vi "PH_gentec_P-Link.ProcPeriodic.vi"(0 "i ref in":refnum<vi>, 3 "ms timeout (100)":i32=100, 5 "error in (no error)":errorcluster) -> (14 "i ref out":refnum<vi>, 17 "timed out":bool, 19 "error out":errorcluster)   [LabVIEW 2014, in "PH_gentec_P-Link.lvlib"]
doc: "This method serves to periodically do things. In this case, it reads the current value from the powermeter. If the Start Stop - value is true, the statistic data is read out as well. Finally, these data is send to own attributes and the GUI elements."
uses:
  PH_gentec_P-Link.lvlib
  PH_Basics/PH_Powermeter_BaseClass/PH_Powermeter_BaseClass.lvlib
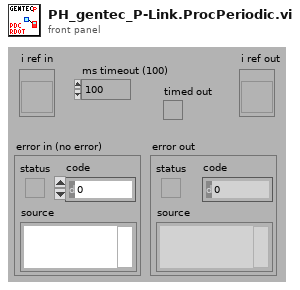
[diagram p1: front panel]
types:
  T1 = typedef "PH_Powermeter_BaseClass.lvlib/PH_Powermeter_BaseClass.State.ctl" = enum32{"off", "operating", "opened", "checked", "connected", "Sets to change", "running"}
  T2 = typedef "PH_gentec_P-Link.lvlib/PH_gentec_P-Link.i attribute.ctl" = cluster{"GUI References":cluster{"Wanted Head Settings":refnum<vi>, "Current Head Settings":refnum<vi>, "Set Auto Range":refnum<vi>, "Trigger Polarity":refnum<vi>, "Trigger Source":refnum<vi>, "Waveform Averages":refnum<vi>, "Continuous":refnum<vi>, "get one Value":refnum<vi>, "Set Zero":refnum<vi>}, "Wanted Head Settings":T3, "Current Head Settings":T3}
  T3 = typedef "PH_gentec_P-Link.lvlib/PH_gentec_P-Link.Head Settings.ctl" = cluster{"Enable Anticipation":bool, "Set Auto Range":bool, "Set Zero":i32, "Current":i32, "Start Data Flow":bool}
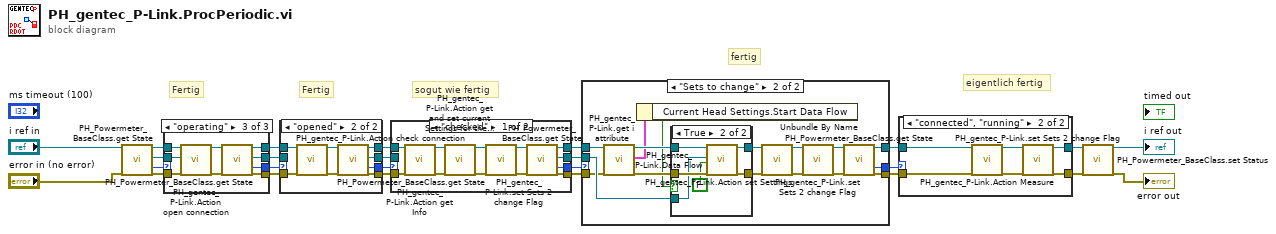
[diagram p0: block diagram]
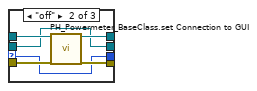
[diagram p8: hidden frame]
diagram:
  # "eigentlich fertig"
  # "fertig"
  # "sogut wie fertig"
  # "Fertig"
  # "Fertig"
  n1 = call "PH_Powermeter_BaseClass.get State.vi"("VI in"="i ref in", "error in (no error)"="error in (no error)") -> ("VI out"=w24:refnum<vi>, "VISA resource"=w23:refnum<visa-resource-name>, "State"=w18:T1, "error out"=w25:errorcluster)  [unwired: 14 in]
  n2 = case shown="\"operating\"" w18 {
    selector: w18 -> [w27 w30 _]
    tunnel: w25 -> [w29 w34 w44]
    tunnel: [w29 w32 w40] -> w16
    tunnel: w23 -> [w28 w31 w43]
    tunnel: [w28 w31 w37] -> w14
    tunnel: [w27 w30 w36] -> w15
    tunnel: w24 -> [w26 w35 w42]
    tunnel: [w26 w33 w38] -> w17
    frame Default {
    }
    frame "off" {
      n3 = call "PH_Powermeter_BaseClass.set Connection to GUI.vi"("i ref in"=w35, "error in"=w34) -> ("i ref out"=w33:refnum<vi>, "error out"=w32:errorcluster)  [unwired: 16 in]
    }
    frame "operating" {
      n4 = call "PH_gentec_P-Link.Action open connection.vi"("i ref in"=w42, "VISA resource in"=w43, "error in"=w44) -> ("i ref out"=w39:refnum<vi>, "error out"=w41:errorcluster)  [unwired: 15 in]
      n5 = call "PH_Powermeter_BaseClass.get State.vi"("VI in"=w39, "error in (no error)"=w41) -> ("VI out"=w38:refnum<vi>, "VISA resource"=w37:refnum<visa-resource-name>, "State"=w36:T1, "error out"=w40:errorcluster)  [unwired: 14 in]
    }
  }
  n6 = case shown="\"opened\"" w15 {
    selector: w15 -> [w46 _]
    tunnel: w16 -> [w48 w49]
    tunnel: [w48 w54] -> w12
    tunnel: w14 -> [w47 _]
    tunnel: [w47 w51] -> w10
    tunnel: [w46 w50] -> w11
    tunnel: w17 -> [w45 w56]
    tunnel: [w45 w52] -> w13
    frame Default {
    }
    frame "opened" {
      n7 = call "PH_gentec_P-Link.Action check connection.vi"("i ref in"=w56, "error in"=w49) -> ("i ref out"=w53:refnum<vi>, "error out"=w55:errorcluster)  [unwired: 16 in]
      n8 = call "PH_Powermeter_BaseClass.get State.vi"("VI in"=w53, "error in (no error)"=w55) -> ("VI out"=w52:refnum<vi>, "VISA resource"=w51:refnum<visa-resource-name>, "State"=w50:T1, "error out"=w54:errorcluster)  [unwired: 14 in]
    }
  }
  n9 = case shown="\"checked\"" w11 {
    selector: w11 -> [_ w69]
    tunnel: w13 -> [w68 w72]
    tunnel: w12 -> [w67 w71]
    tunnel: [w66 w72] -> w4
    tunnel: [w65 w71] -> w3
    tunnel: w10 -> [_ w70]
    tunnel: [w64 w70] -> w6
    tunnel: [w63 w69] -> w2
    frame "checked" {
      n10 = call "PH_gentec_P-Link.Action get Info.vi"("i ref in"=w68, "error in"=w67) -> ("i ref out"=w60:refnum<vi>, "error out"=w59:errorcluster)  [unwired: 16 in]
      n11 = call "PH_gentec_P-Link.Action get and set current Settings for the first Time.vi"("i ref in"=w60, "error in"=w59) -> ("i ref out"=w58:refnum<vi>, "error out"=w57:errorcluster)  [unwired: 16 in]
      n12 = call "PH_gentec_P-Link.set Sets 2 change Flag.vi"("i ref in"=w58, "error in"=w57) -> ("i ref out"=w62:refnum<vi>, "error out"=w61:errorcluster)  [unwired: 16 in]
      n13 = call "PH_Powermeter_BaseClass.get State.vi"("VI in"=w62, "error in (no error)"=w61) -> ("VI out"=w66:refnum<vi>, "VISA resource"=w64:refnum<visa-resource-name>, "State"=w63:T1, "error out"=w65:errorcluster)  [unwired: 14 in]
    }
    frame Default {
    }
  }
  n14 = case shown="\"Sets to change\"" w2 {
    selector: w2 -> [w73 _]
    tunnel: [w75 w89] -> w7
    tunnel: w6 -> [_ w88]
    tunnel: [w74 w87] -> w5
    tunnel: w4 -> [w75 w85]
    tunnel: w3 -> [w74 w83]
    tunnel: [w73 w80] -> w1
    frame Default {
    }
    frame "Sets to change" {
      n15 = call "PH_gentec_P-Link.get i attribute.vi"("i ref in"=w85, "error in (no error)"=w83) -> ("i ref out"=w86:refnum<vi>, "i attribute"=w82:T2, "error out"=w84:errorcluster)  [unwired: 15 in]
      n16 = Unbundle By Name(w82) -> ("Current Head Settings.Start Data Flow"=w81:bool)
      n17 = case shown="True" w81 {
        tunnel: w84 -> [w92 w99]
        tunnel: [w92 w98] -> w91
        tunnel: w86 -> [w93 w97]
        tunnel: [w93 w96] -> w90
        tunnel: w88 -> [_ w95]
        frame False {
        }
        frame True {
          n18 = call "PH_gentec_P-Link.Data Flow.vi"("i ref in"=w97, "VISA resource in"=w95, "Data Flow State to set"=FALSE, "error in"=w99) -> ("i ref out"=w96:refnum<vi>, "error out"=w98:errorcluster)  [unwired: 10 in, 4 out]
        }
      }
      n19 = call "PH_gentec_P-Link.Action set Settings.vi"("i ref in"=w90, "error in"=w91) -> ("i ref out"=w77:refnum<vi>, "error out"=w76:errorcluster)  [unwired: 16 in]
      n20 = call "PH_gentec_P-Link.set Sets 2 change Flag.vi"("i ref in"=w77, "error in"=w76) -> ("i ref out"=w79:refnum<vi>, "error out"=w78:errorcluster)  [unwired: 16 in]
      n21 = call "PH_Powermeter_BaseClass.get State.vi"("VI in"=w79, "error in (no error)"=w78) -> ("VI out"=w89:refnum<vi>, "State"=w80:T1, "error out"=w87:errorcluster)  [unwired: 14 in, 1 out]
    }
  }
  n22 = case shown="\"connected\", \"running\"" w1 {
    tunnel: [w100 w102] -> w22
    tunnel: [w101 w103] -> w21
    tunnel: w7 -> [w101 w107]
    tunnel: w5 -> [w100 w106]
    frame Default {
    }
    frame "connected", "running" {
      n23 = call "PH_gentec_P-Link.Action Measure.vi"("VI in"=w107, "error in (no error)"=w106) -> ("VI out"=w104:refnum<vi>, "error out"=w105:errorcluster)  [unwired: 16 in]
      n24 = call "PH_gentec_P-Link.set Sets 2 change Flag.vi"("i ref in"=w104, "error in"=w105) -> ("i ref out"=w103:refnum<vi>, "error out"=w102:errorcluster)  [unwired: 16 in]
    }
  }
  n25 = call "PH_Powermeter_BaseClass.set Status.vi"("i ref in"=w21, "error in"=w22) -> ("i ref out"=→"i ref out":refnum<vi>, "error out"=→"error out":errorcluster)  [unwired: 16 in]
